vi "Network stream test.vi"() -> ()   [LabVIEW 2018]
panel:
  out "data out":cluster{"Command":string, "Data":variant}
  out "connectLED":bool caption="Waiting for connection"
  in  "Quit All":bool
  in  "Quit":bool
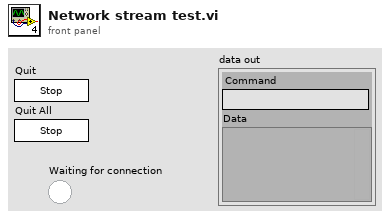
[diagram p1: front panel]
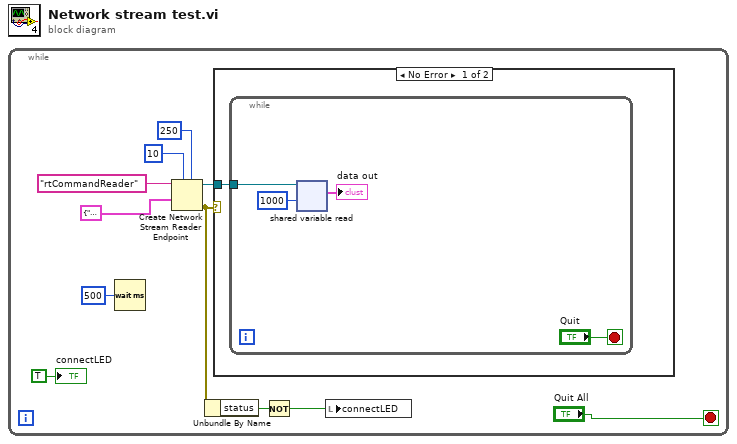
[diagram p0: block diagram]
diagram:
  n1 = while {
    stop <- "Quit All" stop-if-true
    n2 = Wait (ms)(milliseconds to wait=u32 500) -> ()  [unwired: 1 out]
    n3 = Create Network Stream Reader Endpoint(5:250 ("timeout in ms (-1)"), 7:10 ("reader buffer size"), 9:cluster{"Command":string, "Data":variant} {"Command"="", "Data"=variant}, 11:"rtCommandReader" ("reader name")) -> (0:w3:errorcluster, 3:w8:refnum<k21>)  [unwired: 3 in]
    n4 = Unbundle By Name(w3) -> ("status"=w2:bool)
    n5 = case shown="No Error" w3 {
      tunnel: w8 -> [w12 _]
      frame No Error {
        n6 = while {
          tunnel: w12 -> [w15]
          stop <- "Quit" stop-if-true
          n7 = shared-variable-read(w15, 1000 ("timeout ms (-1)")) -> (→"data out":cluster{"Command":string, "Data":variant})  [unwired: 1 in, 3 out]
        }
      }
      frame Error {
      }
    }
    n8 = Not(x=w2) -> (.not. x?=w1:bool)
    n9 = local write "connectLED"(w1) -> ()
    "connectLED" <- TRUE ("connectLED")
  }
